vi "MPXsetAmplitude.vi"(2 "Refresh":bool, 3 "Amplitude [V]":i32=100, 4 "Comport in":refnum<visa-resource-name>="COM5") -> (0 "read buffer":string="boff\r\nSignal off\r\n\r\nWavetype: Sawtooth\r\nFrequence: 0116 Hz\r\nAmplitude: 202,0 V\r\nSignal off\r\n\r\nempc>:\n", 1 "Comport out":refnum<visa-resource-name>="COM5")   [LabVIEW 2015]
uses:
  Instance           1 24Saved   MPX setAmplitude .vi
panel:
  out "Amplitude bkp":i32=100
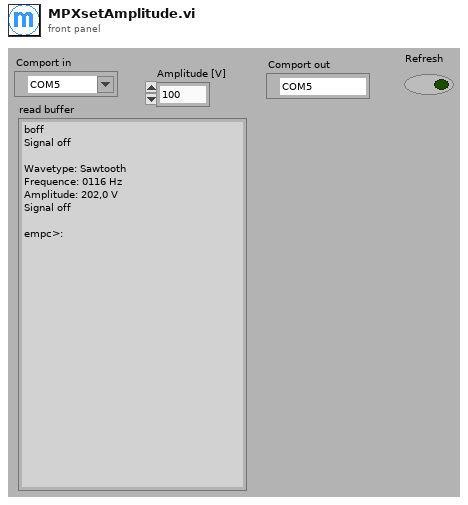
[diagram p1: front panel]
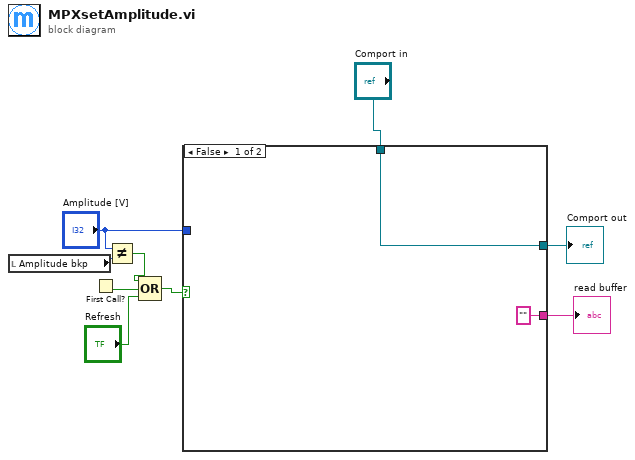
[diagram p0: block diagram]
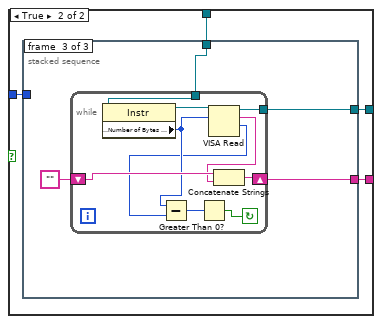
[diagram p2: hidden frame]
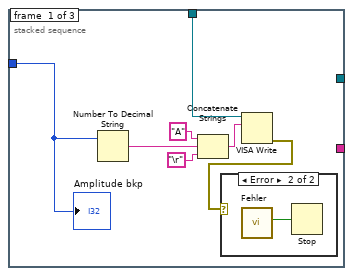
[diagram p3: hidden frame]
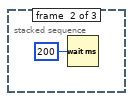
[diagram p5: hidden frame]
diagram:
  n1 = local read "Amplitude bkp"() -> (w4:i32)
  n2 = First Call?() -> (First Call?: T/F=w2:bool)
  n3 = Not Equal?(x="Amplitude [V]", y=w4) -> (x != y?=w3:bool)
  n4 = Compound Arithmetic op=OR(w3, w2, "Refresh") -> (w7:bool)
  n5 = case shown="False" w7 {
    tunnel: "Comport in" -> [w11 w15]
    tunnel: "Amplitude [V]" -> [_ w14]
    tunnel: [w11 w13] -> w8
    tunnel: ["" w12] -> w1
    frame False {
    }
    frame True {
      n6 = stacked-sequence {
        tunnel: w15 -> [w19 _ w28]
        tunnel: w14 -> [w17 _ _]
        tunnel: [_ _ w26] -> w13
        tunnel: [_ _ w25] -> w12
        frame #0 {
          n7 = Number To Decimal String(number=w17) -> (decimal integer string=w18:string)  [unwired: 1 in]
          n8 = Concatenate Strings("A", w18, "\r") -> (w22:string)
          n9 = VISA Write(VISA resource name=w19, write buffer=w22) -> (error out=w16:errorcluster)  [unwired: 1 in, 2 out]
          n10 = case shown="Error" w16 {
            frame No Error {
            }
            frame Error {
              n11 = call "Fehler"() -> ("OK"=w23:bool)  [unwired: 10 in, 1 out]
              n12 = Stop(stop? (T)=w23) -> ()
            }
          }
          "Amplitude bkp" <- w17
        }
        frame #1 {
          n13 = Wait (ms)(milliseconds to wait=u32 200) -> ()  [unwired: 1 out]
        }
        frame #2 {
          n14 = while {
            shift-right: [w36] -> w25
            shift-left: "" -> [w37]
            tunnel: w28 -> [w30]
            tunnel: [w29] -> w26
            stop <- w31 continue-if-true
            n15 = property class="Instr"(reference=w30) -> (reference out=w38:refnum<visa-resource-name>, "Serial Settings:Number of Bytes at Serial Port"=w33:u32)  [unwired: 1 in, 1 out]
            n16 = VISA Read(VISA resource name=w38, byte count=w33) -> (VISA resource name out=w29:refnum<visa-resource-name>, read buffer=w35:string, return count=w32:u32)  [unwired: 1 in, 1 out]
            n17 = Subtract(x=w33, y=w32) -> (x-y=w34:u32)
            n18 = Greater Than 0?(x=w34) -> (x > 0?=w31:bool)
            n19 = Concatenate Strings(w37, w35) -> (w36:string)
          }
        }
      }
    }
  }
  "Comport out" <- w8
  "read buffer" <- w1
